vi "UnlockSurface.vi"(8 "No Error":errorcluster, 11 "Surface [SDL_Surface *]":i64 format="%.0x") -> (0 "error out":errorcluster)   [LabVIEW 2024, in "SDL3.lvlib" / "Surface.lvlib"]
doc: "<B>Summary</B>\nRelease a surface after directly accessing the pixels."
uses:
  Surface.lvlib
  <vilib>/Utility/error.llb/Error Cluster From Error Code.vi
  Error/Error.lvlib
  Lib/Win32/SDL3.dll
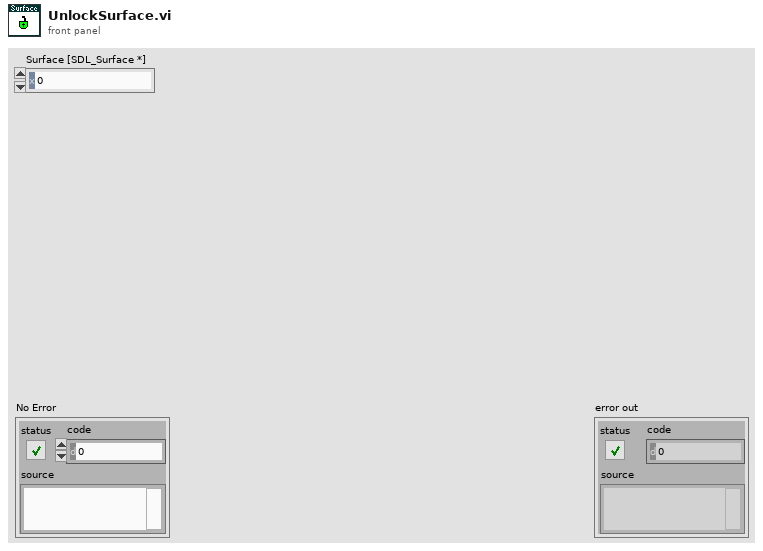
[diagram p1: front panel]
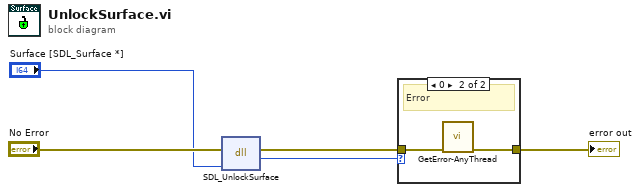
[diagram p0: block diagram]
diagram:
  n1 = dll-call lib="C:/Users/Thomas/Documents/Projects/LV-SDL3/Lib/Win32/SDL3.dll" fn="SDL_UnlockSurface"(error in="No Error", "surface"="Surface [SDL_Surface *]") -> (error out=w2:errorcluster, "return type"=w1:i32)  [unwired: 3 in, 1 out]
  n2 = case shown="0" w1 {
    tunnel: w2 -> [w6 w8]
    tunnel: [w6 w7] -> w4
    frame Default {
      # "Ok"
    }
    frame 0 {
      # "Error"
      n3 = call "GetError-AnyThread.vi"("No Error"=w8) -> ("Error Out"=w7:errorcluster)  [unwired: 10 in]
    }
  }
  "error out" <- w4
